vi "gun_speed_control_feed_forward.vi"(9 "Period (sec)":dbl, 10 "Speed (rps)":dbl, 11 "Gun Const":T2={"gun"={"num_lines"=0.0, "gain_kp1"=0.0, "gain_kp2"=0.0, "gain_ki"=0.0, "gain_kd"=0.0}, "turret"={"center_ana"=0.0, "volts_per_180"=0.0, "man_scale"=0.0, "turret_idg"={"low_fault_ana"=0.0, "high_fault_ana"=0.0, "min_ana"=0.0, "max_ana"=0.0, "movement_thresh"=0.0, "movement_time"=0.0}, "turret_pid"={"kP"=0.0, "kI"=0.0, "kD"=0.0}, "turret_invert"=TRUE, "turret_low_power"=0.0}, "tracking"={"velocity_lead_gain"=0.0, "velocity_rotation_gain"=0.0}, "hood"={"hood_idg"={"low_fault_ana"=0.0, "high_fault_ana"=0.0, "min_ana"=0.0, "max_ana"=0.0, "movement_thresh"=0.0, "movement_time"=0.0}, "hood_pid"={"kP"=0.0, "kI"=0.0, "kD"=0.0}, "hood_scale"={"min_ana"=0.0, "min_units"=0.0, "max_ana"=0.0, "max_units"=0.0}, "hood_invert"=FALSE}}) -> (1 "rpm raw":dbl, 2 "Sensor Speed (rps)":dbl, 3 "Output":dbl)   [LabVIEW 2011]
uses:
  gun_const_t.ctl
  gun_idg_const.ctl
  common/gain_const.ctl
  common/scale_const.ctl
  signals/Signal.ctl
  <vilib>/ptbypt/NI_PtbyPt.lvlib
  <vilib>/Analysis/3filter.llb/Filter Passband Type.ctl
  <vilib>/Analysis/NI_AALBase.lvlib
panel:
  in  "Scale Const":T1={"min_ana"=0.0, "min_units"=1.0, "max_ana"=400.0, "max_units"=0.0}
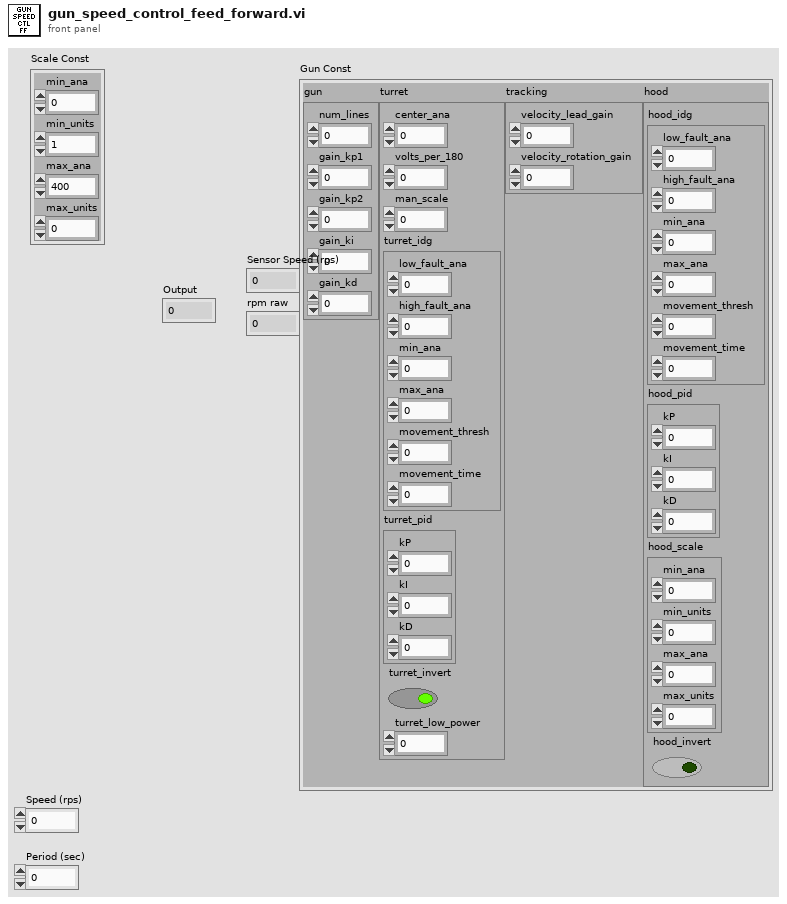
[diagram p1: front panel]
types:
  T1 = typedef "scale_const.ctl" = cluster{"min_ana":dbl, "min_units":dbl, "max_ana":dbl, "max_units":dbl}
  T2 = typedef "gun_const_t.ctl" = cluster{"gun":cluster{"num_lines":dbl, "gain_kp1":dbl, "gain_kp2":dbl, "gain_ki":dbl, "gain_kd":dbl}, "turret":cluster{"center_ana":dbl, "volts_per_180":dbl, "man_scale":dbl, "turret_idg":T3, "turret_pid":T4, "turret_invert":bool, "turret_low_power":dbl}, "tracking":cluster{"velocity_lead_gain":dbl, "velocity_rotation_gain":dbl}, "hood":cluster{"hood_idg":T3, "hood_pid":T4, "hood_scale":T1, "hood_invert":bool}}
  T3 = typedef "gun_idg_const.ctl" = cluster{"low_fault_ana":dbl, "high_fault_ana":dbl, "min_ana":dbl, "max_ana":dbl, "movement_thresh":dbl, "movement_time":dbl}
  T4 = typedef "gain_const.ctl" = cluster{"kP":dbl, "kI":dbl, "kD":dbl}
  T5 = typedef "Signal.ctl" = enum16{"SIGFIRE", "SIGSTOPSCRIPT", "SIGSTARTGUN", "SIGSTOPGUN", "SIGDISABLED", "SIGENABLED", "SIGUDPTIMEOUT", "SIGNEWVISION_REMOTE", "SIGNEWVISION_LOCAL", "SIGSHOTFIRED", "SIGDOTRACK", "SIGDONTTRACK"}
  T6 = typedef "NI_AALBase.lvlib/Filter Passband Type.ctl" = enum32{"Lowpass", "Highpass", "Bandpass", "Bandstop"}
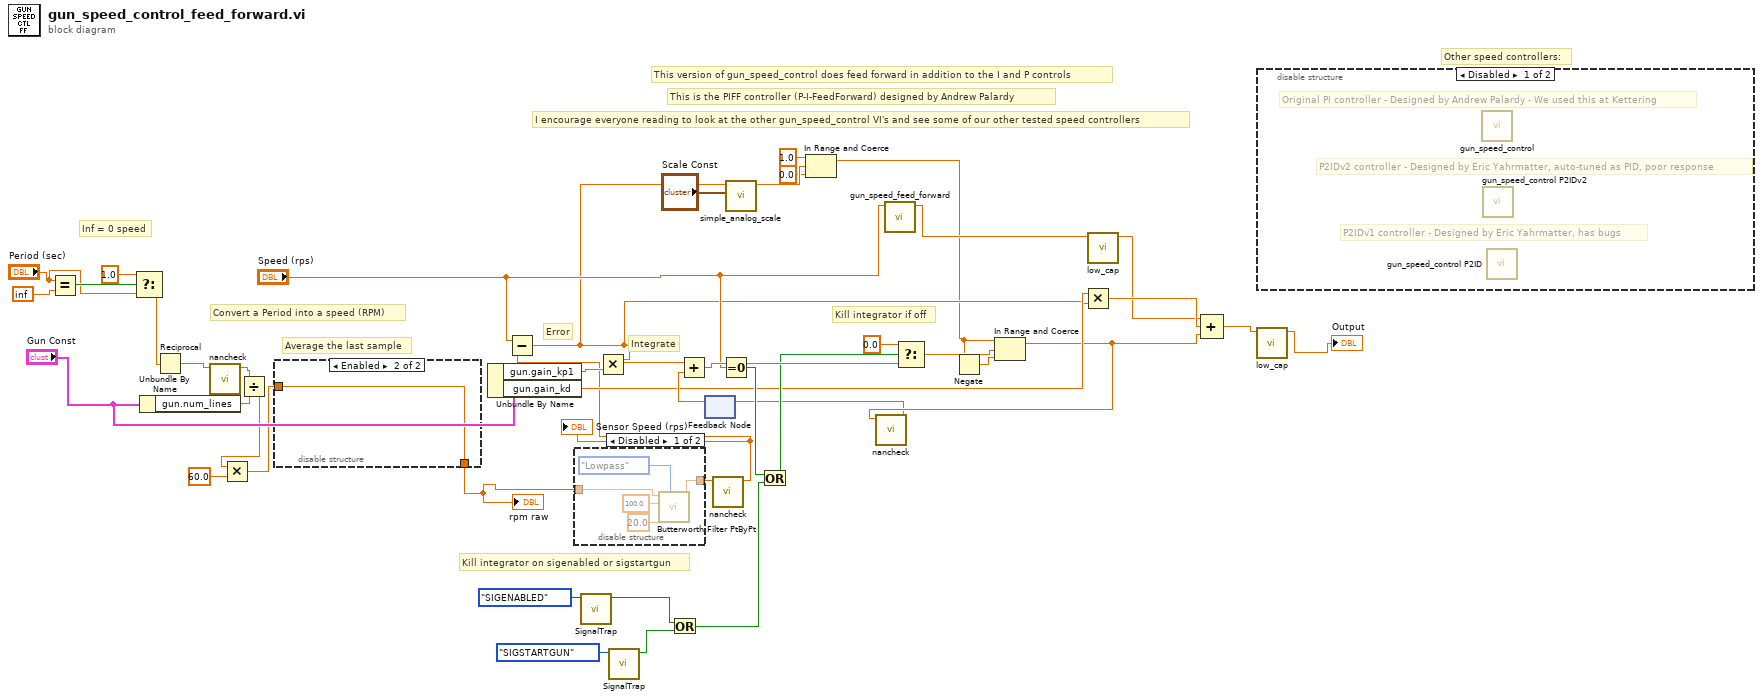
[diagram p0: block diagram]
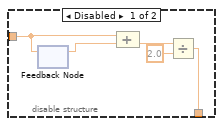
[diagram p4: hidden frame]
diagram:
  # "This is the PIFF controller (P-I-FeedForward) designed by Andrew Palardy"
  # "Other speed controllers:"
  # "I encourage everyone reading to look at the other gun_speed_control VI's and see some of our other tested speed controllers"
  # "This version of gun_speed_control does feed forward in addition to the I and P controls"
  # "Inf = 0 speed"
  # "Kill integrator on sigenabled or sigstartgun"
  # "Average the last sample"
  # "Kill integrator if off"
  # "Integrate"
  # "Error"
  # "Convert a Period into a speed (RPM)"
  n1 = Equal?(x="Period (sec)", y=inf) -> (x = y?=w32:bool)
  n2 = Select(t=1.0, s=w32, f="Period (sec)") -> (s? t:f=w21:dbl)
  n3 = Unbundle By Name("Gun Const") -> ("gun.num_lines"=w43:dbl)
  n4 = Reciprocal(x=w21) -> (1/x=w22:dbl)
  n5 = call "nancheck.vi"("nancheck_in"=w22) -> ("nancheck_out"=w23:dbl)  [unwired: 10 in]
  n6 = Divide(x=w23, y=w43) -> (x/y=w14:dbl)
  n7 = Multiply(x=w14, y=60.0) -> (x*y=w15:dbl)
  n8 = disable-structure shown="Enabled" {
    disable-tunnel: w15 -> [w46 w50]
    disable-tunnel: [w45 w50] -> w16
    frame Disabled {
      n9 = feedback #1() -> (w47:dbl)  [unwired: 1 in]
      n10 = feedback-in #1(w46) -> ()
      n11 = Compound Arithmetic op=ADD(w46, w47) -> (w48:dbl)
      n12 = Divide(x=w48, y=2.0) -> (x/y=w45:dbl)
    }
    frame Enabled {
    }
  }
  "rpm raw" <- w16
  n13 = Unbundle By Name("Gun Const") -> ("gun.gain_kp1"=w44:dbl, "gun.gain_kd"=w28:dbl)
  n14 = disable-structure shown="Disabled" {
    disable-tunnel: w16 -> [w52 w56]
    disable-tunnel: [w51 w56] -> w24
    frame Disabled {
      n15 = call <vilib>:"Butterworth Filter PtByPt.vi"("filter type"=Filter_Passband_Type."Lowpass", "low cutoff freq: fl"=20.0, "sampling freq: fs"=100.0, "x"=w52) -> ("Filtered x"=w51:dbl)  [unwired: 5 in, 1 out]
    }
    frame Enabled {
    }
  }
  n16 = call "SignalTrap.vi"("Signal"=Signal."SIGENABLED") -> ("Trapped Signal"=w19:bool)  [unwired: 10 in]
  n17 = call "SignalTrap.vi"("Signal"=Signal."SIGSTARTGUN") -> ("Trapped Signal"=w18:bool)  [unwired: 10 in]
  n18 = Or(x=w19, y=w18) -> (x .or. y?=w17:bool)
  n19 = feedback #2() -> (w40:dbl)  [unwired: 1 in]
  n20 = call "nancheck.vi"("nancheck_in"=w24) -> ("nancheck_out"=w25:dbl)  [unwired: 10 in]
  "Sensor Speed (rps)" <- w25
  n21 = Subtract(x="Speed (rps)", y=w25) -> (x-y=w7:dbl)
  n22 = Multiply(x=w7, y=w44) -> (x*y=w39:dbl)
  n23 = Add(x=w39, y=w40) -> (x+y=w41:dbl)
  n24 = Equal To 0?(x="Speed (rps)") -> (x = 0?=w35:bool)
  n25 = call "simple_analog_scale.vi"("Scale Const"="Scale Const", "Analog"=w7) -> ("Units"=w5:dbl)  [unwired: 9 in]
  n26 = Or(x=w35, y=w17) -> (x .or. y?=w34:bool)
  n27 = In Range and Coerce(upper limit=1.0, x=w5, lower limit=0.0) -> (coerced(x)=w3:dbl)  [unwired: 1 out]
  n28 = call "gun_speed_feed_forward.vi"("RPM"="Speed (rps)") -> ("Power"=w8:dbl)  [unwired: 10 in]
  n29 = Select(t=0.0, s=w34, f=w41) -> (s? t:f=w37:dbl)
  n30 = Negate(x=w3) -> (-x=w6:dbl)
  n31 = In Range and Coerce(upper limit=w3, x=w37, lower limit=w6) -> (coerced(x)=w27:dbl)  [unwired: 1 out]
  n32 = call "nancheck.vi"("nancheck_in"=w27) -> ("nancheck_out"=w26:dbl)  [unwired: 10 in]
  n33 = feedback-in #2(w26) -> ()
  n34 = Multiply(x=w28, y=w7) -> (x*y=w29:dbl)
  n35 = call "low_cap.vi"("num"=w8) -> ("lim"=w12:dbl)  [unwired: 10 in]
  n36 = Compound Arithmetic op=ADD(w12, w29, w27) -> (w11:dbl)
  n37 = call "low_cap.vi"("num"=w11) -> ("lim"=→"Output":dbl)  [unwired: 10 in]
  n38 = disable-structure shown="Disabled" {
    frame Disabled {
      # "P2IDv1 controller - Designed by Eric Yahrmatter, has bugs"
      # "P2IDv2 controller - Designed by Eric Yahrmatter, auto-tuned as PID, poor response"
      # "Original PI controller - Designed by Andrew Palardy - We used this at Kettering"
      n39 = call "gun_speed_control.vi"() -> ()  [unwired: 9 in, 3 out]
      n40 = call "gun_speed_control P2IDv2.vi"() -> ()  [unwired: 9 in, 3 out]
      n41 = call "gun_speed_control P2ID.vi"() -> ()  [unwired: 9 in, 3 out]
    }
    frame Enabled {
    }
  }
